vi "ICM List Scaling Instances.vi"(8 "error in (no error)":errorcluster, 11 "Scalings":string[](array[string])) -> (0 "error out":errorcluster, 3 "Instances":cluster{"Instances":string[]}[](array[cluster]))   [LabVIEW 2024]
doc: "ICM List Scaling Instances.vi\n\nThis VI creates a list of all the scaling \"instances\" that exist in the current configuration file. It also creates a parallel array which names the Scaling child class of each instance.\n\nInstrument Communication Module Version 1.0\nSeptember, 2017 Original Code Consulting David Thomson\n www.originalcode.com"
uses:
  Scaling/Scaling.lvclass
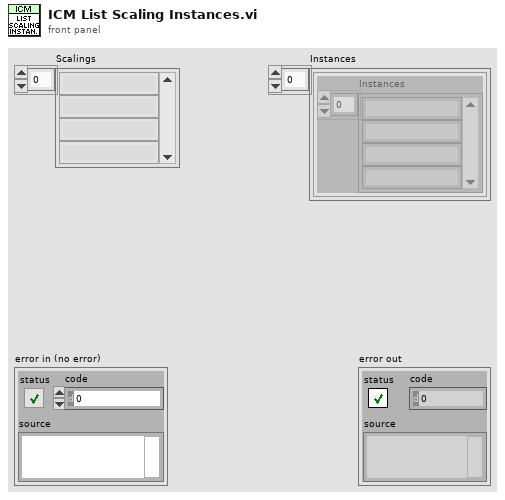
[diagram p1: front panel]
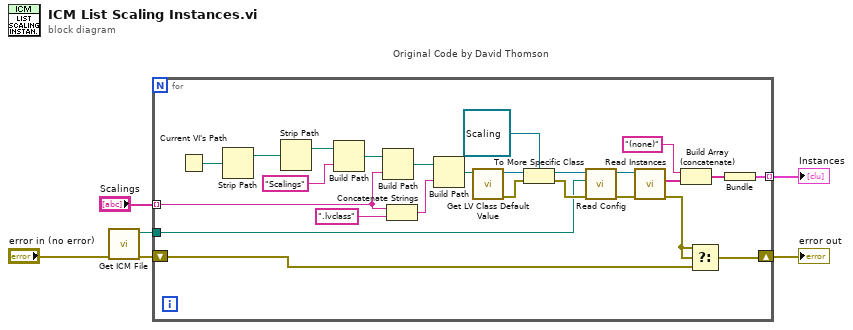
[diagram p0: block diagram]
diagram:
  n1 = call "Get ICM File.vi"("error in (no error)"="error in (no error)") -> ("error out"=w4:errorcluster, "ICM File"=w3:path)  [unwired: 9 in]
  n2 = for "Original Code by David Thomson" {
    tunnel: "Scalings" -> [w13] mode=indexing
    shift-right: [w15] -> w2
    shift-left: w4 -> [w14]
    tunnel: w3 -> [w19]
    tunnel: [w12] -> w1 mode=indexing
    n3 = Current VI's Path() -> (path=w10:path)
    n4 = Strip Path(path=w10) -> (stripped path=w11:path)  [unwired: 1 out]
    n5 = Strip Path(path=w11) -> (stripped path=w29:path)  [unwired: 1 out]
    n6 = Build Path(base path=w29, name or relative path="Scalings") -> (appended path=w30:path)
    n7 = Build Path(base path=w30, name or relative path=w13) -> (appended path=w27:path)
    n8 = Concatenate Strings(w13, ".lvclass" ("string")) -> (w25:string)
    n9 = Build Path(base path=w27, name or relative path=w25) -> (appended path=w28:path)
    n10 = call <vilib>:"Get LV Class Default Value.vi"("class path"=w28) -> ("error out"=w24:errorcluster, "object"=w23:refnum<class>)  [unwired: 9 in]
    n11 = To More Specific Class(target class=refnum<class "Scaling.lvclass"> refnum ("Scaling.lvclass"), reference=w23, error in=w24) -> (specific class reference=w20:refnum<class "Scaling.lvclass">, error out=w21:errorcluster)
    n12 = call-dynamic "Read Config.vi"("error in (no error)"=w21, "ICM File In"=w19, "Scaling in"=w20) -> ("error out"=w17:errorcluster, "Scaling out"=w18:refnum<class "Scaling.lvclass">)  [unwired: 7 in]
    n13 = call-dynamic "Read Instances.vi"("error in (no error)"=w17, "Scaling in"=w18) -> ("error out"=w16:errorcluster, "Scaling Instances"=w9:string[])  [unwired: 7 in, 1 out]
    n14 = Build Array (concatenate)("(none)", w9) -> (w8:string[])
    n15 = Select(t=w16, s=w16, f=w14) -> (s? t:f=w15:errorcluster)
    n16 = Bundle(w8) -> (w12:cluster{string[]})  [unwired: 1 in]
  }
  "error out" <- w2
  "Instances" <- w1
